vi "makeDecisions.vi"(8 "error in (no error)":errorcluster, 10 "model":refnum<class "Model.lvclass">, 11 "RampingUpPressurePState in":refnum<class "RampingUpPressurePState.lvclass">) -> (0 "error out":errorcluster, 2 "model 2":refnum<class "Model.lvclass">, 3 "RampingUpPressurePState out":refnum<class "RampingUpPressurePState.lvclass">)   [LabVIEW 2015, in "RampingUpPressurePState.lvclass"]
uses:
  RampingUpPressurePState.lvclass
  Model/Model/Model.lvclass
  Typedefs/StateSelector.ctl
  PreconditioningState/PreconditioningState.lvclass
  Typedefs/M1M3SSSTypedefs.lvlib
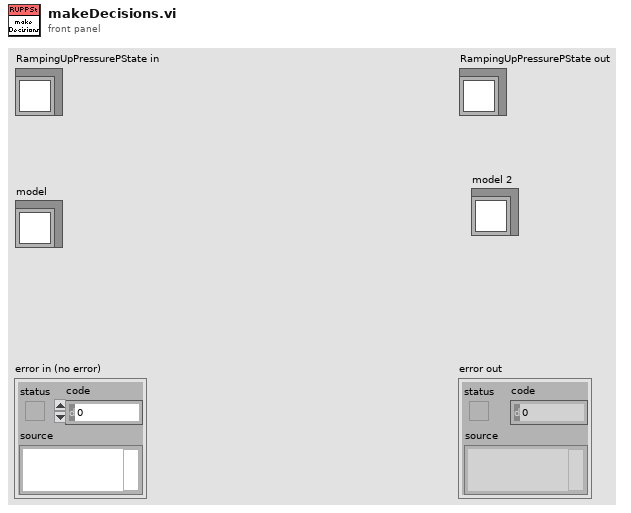
[diagram p1: front panel]
types:
  T1 = typedef "M1M3SSSTypedefs.lvlib/StateSelector.ctl" = enum16{"FaultState", "OffState", "RampingUpPressurePState", "RampingUpPressureSTState", "StandbyState", "StoppedState", "WaitingForSettledPState", "WaitingForSettledSTState"}
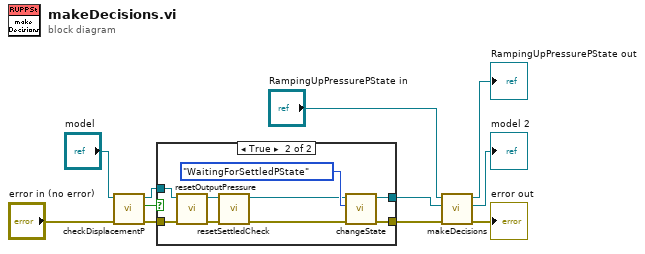
[diagram p0: block diagram]
diagram:
  n1 = call "checkDisplacementP.vi"("error in (no error)"="error in (no error)", "Model in"="model") -> ("error out"=w4:errorcluster, "reachedDisplacementTriggerIsTrue"=w6:bool, "Model out"=w5:refnum<class "Model.lvclass">)  [unwired: 7 in]
  n2 = case shown="True" w6 {
    tunnel: w5 -> [w13 w19]
    tunnel: w4 -> [w12 w18]
    tunnel: [w12 w22] -> w3
    tunnel: [w13 w21] -> w1
    frame False {
    }
    frame True {
      n3 = call "resetOutputPressure.vi"("error in (no error)"=w18, "Model in"=w19) -> ("error out"=w16:errorcluster, "Model out"=w17:refnum<class "Model.lvclass">)  [unwired: 8 in]
      n4 = call "resetSettledCheck.vi"("error in (no error)"=w16, "Model in"=w17) -> ("error out"=w14:errorcluster, "Model out"=w15:refnum<class "Model.lvclass">)  [unwired: 7 in, 1 out]
      n5 = call "changeState.vi"("error in (no error)"=w14, "State:"=StateSelector."WaitingForSettledPState", "Model in"=w15) -> ("error out"=w22:errorcluster, "Model out"=w21:refnum<class "Model.lvclass">)  [unwired: 7 in]
    }
  }
  n6 = call-parent "makeDecisions.vi"("error in (no error)"=w3, "model"=w1, "EnabledState in"="RampingUpPressurePState in") -> ("error out"=→"error out":errorcluster, "model 2"=→"model 2":refnum<class "Model.lvclass">, "EnabledState out"=→"RampingUpPressurePState out":refnum<class "RampingUpPressurePState.lvclass">)  [unwired: 6 in]
